vi "Timer_HasPeriodPassed.vi"(8 "Pass_Through_Time":dbl=-1.0 format="%33.4f", 9 "Period":dbl, 11 "in Timer":T1 {"Accumulated TIme" format="%13.5p"; "StartTime" format="%13.5p"}) -> (1 "Expired":bool, 2 "CurrentTImer":dbl, 3 "out Timer":T1 {"Accumulated TIme" format="%13.5p"; "StartTime" format="%13.5p"})   [LabVIEW 2019, in "Trajectory_Library.lvlib"]
doc: "Check if the period specified has passed and if it has, advance the start time by that period. This is useful to decide if it's time to do periodic work without drifting later by the time it took to get around to checking.\n\nInputs:\n - Timer -- The Timer data cluster\n - period -- The period to check for (in seconds).\n\nOutputs:\n - Timer -- The modified Timer data cluster\n - CurrentTimer -- Current time value for this timer in seconds\n - Expired -- True if the period has passed."
uses:
  Trajectory_Library.lvlib
  TypeDef/TIMER.ctl
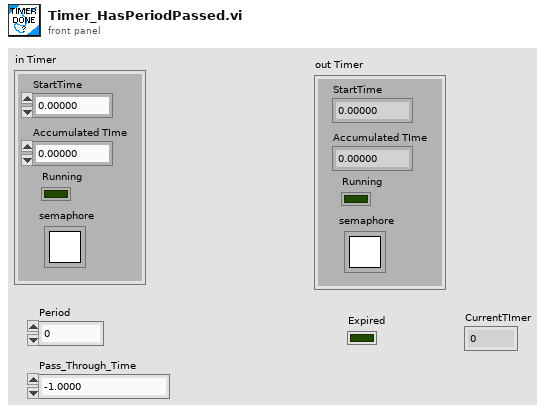
[diagram p1: front panel]
types:
  T1 = typedef "Trajectory_Library.lvlib/TIMER.ctl" = cluster{"StartTime":dbl, "Accumulated TIme":dbl, "Running":bool, "semaphore":T2}
  T2 = typedef "Semaphore RefNum" = refnum<k1>
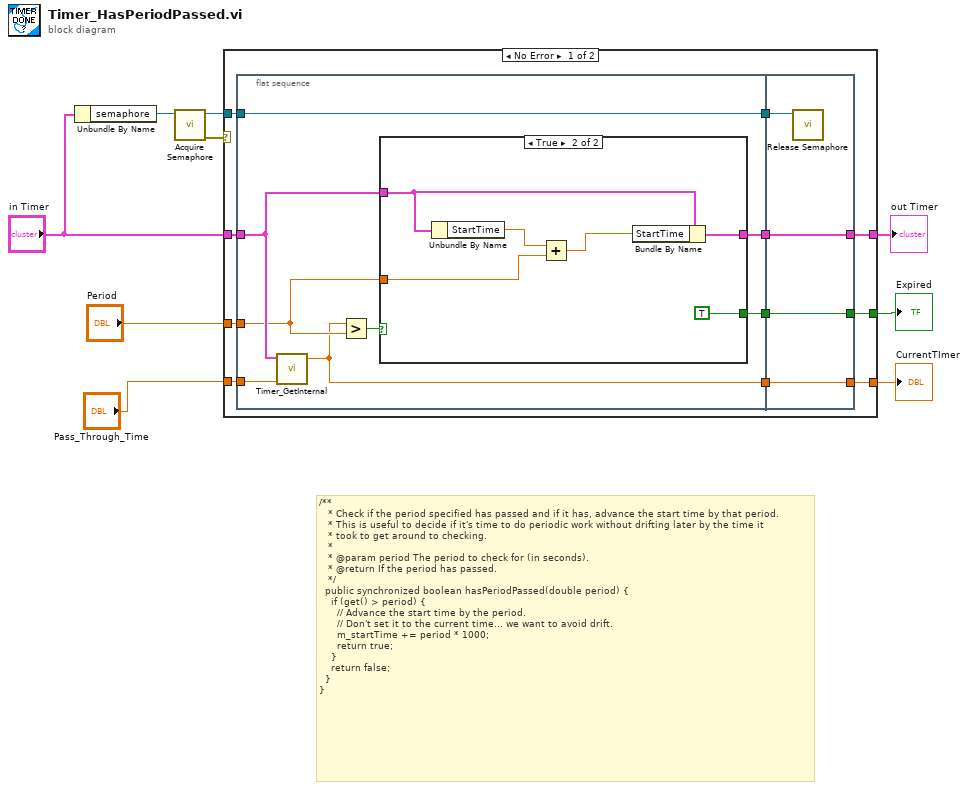
[diagram p0: block diagram]
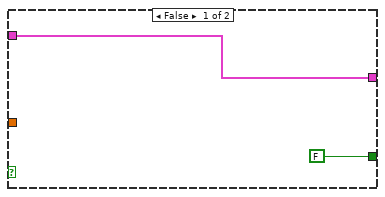
[diagram p2: hidden frame]
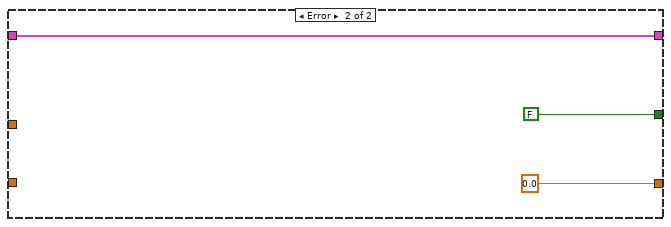
[diagram p3: hidden frame]
diagram:
  # "/**\n   * Check if the period specified has passed and if it has, advance the start time by that period.\n   * This is useful to decide if it's time to do periodic work without drifting later by the time it\n   * took to get around to checking.\n   *\n   * @param period The period to check for (in seconds).\n   * @return If the period has passed.\n   */\n  public synchronized boolean hasPeriodPassed(double period) {\n    if (get() > period) {\n      // Advance the start time by the period.\n      // Don't set it to the current time... we want to avoid drift.\n      m_startTime += period * 1000;\n      return true;\n    }\n    return false;\n  }\n}"
  n1 = Unbundle By Name("in Timer") -> ("semaphore"=w5:T2)
  n2 = call <vilib>:"Acquire Semaphore.vi"("semaphore"=w5) -> ("error out"=w4:errorcluster, "semaphore out"=w3:T2)  [unwired: 4 in, 1 out]
  n3 = case shown="No Error" w4 {
    tunnel: "in Timer" -> [w20 w43]
    tunnel: [w19 w43] -> w9
    tunnel: [w18 FALSE] -> w8
    tunnel: "Period" -> [w17 _]
    tunnel: w3 -> [w11 _]
    tunnel: [w16 0.0 ("CurrentTImer")] -> w2
    tunnel: "Pass_Through_Time" -> [w10 _]
    frame No Error {
      n4 = flat-sequence {
        tunnel: w20 -> [w27]
        tunnel: w17 -> [w24]
        tunnel: [w26] -> w15
        tunnel: [w25] -> w14
        tunnel: [w23] -> w13
        tunnel: [w22] -> w12
        tunnel: w11 -> [w22]
        tunnel: w10 -> [w21]
        tunnel: [w38] -> w16
        tunnel: [w39] -> w18
        tunnel: [w40] -> w19
        tunnel: w15 -> [w40]
        tunnel: w14 -> [w39]
        tunnel: w13 -> [w38]
        tunnel: w12 -> [w37]
        frame #0 {
          n5 = call "Timer_GetInternal.vi"("Pass_Through_Time"=w21, "TIMER"=w27) -> ("CurrentTImer"=w23:dbl)  [unwired: 8 in, 1 out]
          n6 = Greater?(x=w23, y=w24) -> (0:w28:bool)
          n7 = case shown="True" w28 {
            tunnel: w27 -> [w30 w36]
            tunnel: [w30 w35] -> w26
            tunnel: [FALSE TRUE] -> w25
            tunnel: w24 -> [_ w32]
            frame False {
            }
            frame True {
              n8 = Unbundle By Name(w36) -> ("StartTime"=w31:dbl)
              n9 = Add(x=w31, y=w32) -> (x+y=w33:dbl)
              n10 = Bundle By Name(cluster=w36, "StartTime"=w33) -> (w35:T1)
            }
          }
        }
        frame #1 {
          n11 = call <vilib>:"Release Semaphore.vi"("semaphore"=w37) -> ()  [unwired: 5 in, 2 out]
        }
      }
    }
    frame Error {
    }
  }
  "out Timer" <- w9
  "Expired" <- w8
  "CurrentTImer" <- w2
